vi "Peak_Detector.vi"(10 "Data in":waveform(dbl)[](array[waveform]), 11 "Referencia":T1[][](array[typedef])) -> (3 "Detected peaks":T1[][](array[typedef]))   [LabVIEW 2021]
uses:
  Typedefs/Detected peaks.ctl
  <vilib>/measure/matone.llb/Extract Single Tone Information 1 Chan.vi
  <vilib>/measure/NI_MAPro.lvlib
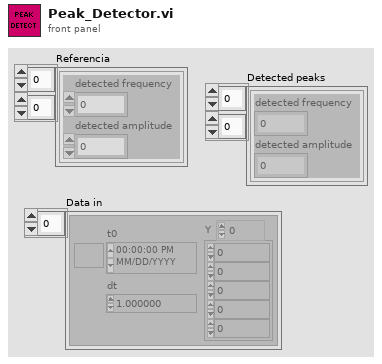
[diagram p1: front panel]
types:
  T1 = typedef "Detected peaks.ctl" = cluster{"detected frequency":dbl, "detected amplitude":dbl}
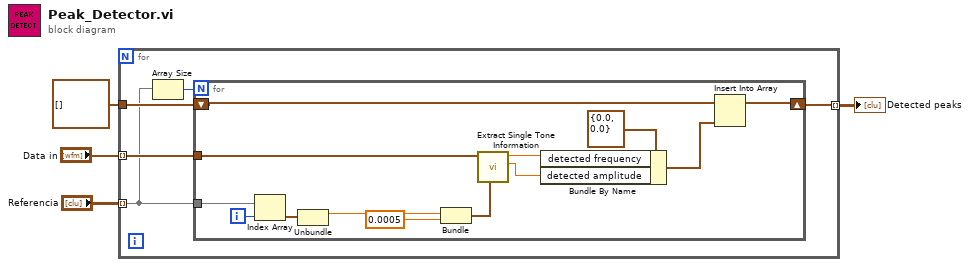
[diagram p0: block diagram]
diagram:
  n1 = for {
    tunnel: "Data in" -> [w9] mode=indexing
    tunnel: "Referencia" -> [w5] mode=indexing
    tunnel: T1[] [] -> [w8]
    tunnel: [w7] -> w3 mode=indexing
    n2 = Array Size(array=w5) -> (size(s)=w6:i32)
    n3 = for {
      N: w6 -> [_]
      tunnel: w9 -> [w22]
      tunnel: w5 -> [w21]
      shift-right: [w11] -> w7
      shift-left: w8 -> [w12]
      i -> [w20]
      n4 = Index Array(array=w21, index=w20) -> (element=w16:T1)
      n5 = Unbundle(w16) -> ("detected frequency"=w14:dbl)  [unwired: 1 out]
      n6 = Bundle("detected frequency"=w14, 0.0005) -> (w13:cluster{"detected frequency":dbl, dbl})  [unwired: 1 in]
      n7 = call-poly <vilib>:"Extract Single Tone Information.vi"("advanced search"=w13, "time signal in"=w22) -> ("detected amplitude"=w18:dbl, "detected frequency"=w19:dbl)  [unwired: 4 in, 4 out]
      n8 = Bundle By Name(cluster=T1 {"detected frequency"=0.0, "detected amplitude"=0.0}, "detected frequency"=w19, "detected amplitude"=w18) -> (w10:T1)
      n9 = Insert Into Array(array=w12, new element=w10) -> (w11:T1[])  [unwired: 1 in]
    }
  }
  "Detected peaks" <- w3
